vi "G#BaseClass1_IG#BaseInterface_Create.vi"(0 "reference in":refnum<class "G#Object.lvclass">, 5 "error in (no error)":errorcluster) -> (14 "reference out":refnum<class "G#BaseClass1_IG#BaseInterface.lvclass">, 19 "error out":errorcluster)   [LabVIEW 2017, in "G#BaseClass1_IG#BaseInterface.lvclass"]
doc: "Creates the interface for the G#Object."
uses:
  G#BaseClass1_IG#BaseInterface.lvclass
  C:/Projects/GsharpGIT2017/Verification/TestCases/TestClasses/IG#BaseInterface_interface/IG#BaseInterface.lvclass
  <vilib>/addons/_AddQ/G#Object/G#Object.lvclass
  IG#BaseInterface_interface/IG#BaseInterface.lvclass
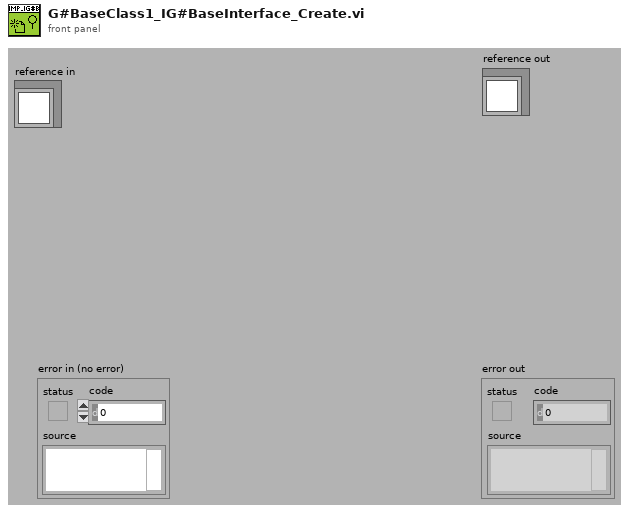
[diagram p1: front panel]
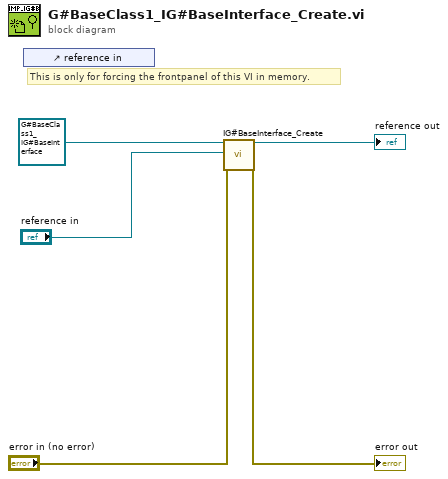
[diagram p0: block diagram]
diagram:
  # "This is only for forcing the frontpanel of this VI in memory."
  n1 = control-ref of="reference in"() -> ()  [unwired: 1 out]
  n2 = call "IG#BaseInterface_Create.vi"("reference in"=refnum<class "G#BaseClass1_IG#BaseInterface.lvclass"> refnum ("reference out"), "G#Object in"="reference in", "error in (no error)"="error in (no error)") -> ("reference out"=→"reference out":refnum<class "G#BaseClass1_IG#BaseInterface.lvclass">, "error out"=→"error out":errorcluster)  [unwired: 15 in]
